vi "camMain - Copy.vi"() -> ()   [LabVIEW 2018]
uses:
  State control.ctl
  <vilib>/userdefined/High Color/IMAQdx.ctl
panel:
  out "Image":T1(plugin-control)
  in  "stop":bool
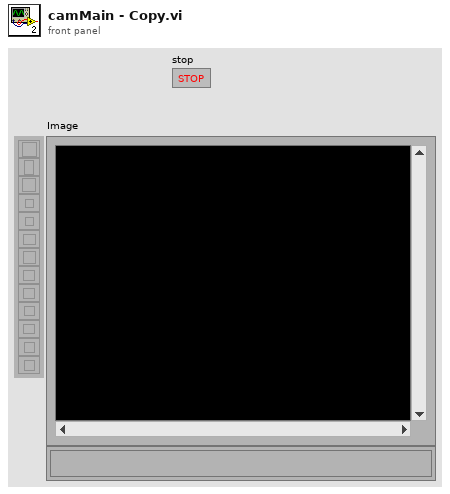
[diagram p1: front panel]
types:
  T1 = typedef "IMAQ Image.ctl" = refnum<image>
  T2 = typedef "IMAQdx.ctl" = refnum<k21>
  T3 = typedef "State control.ctl" = enum16{"Initialise", "Start camera", "Continuous Acquisition ", "Stop camera", "Dispose all"}
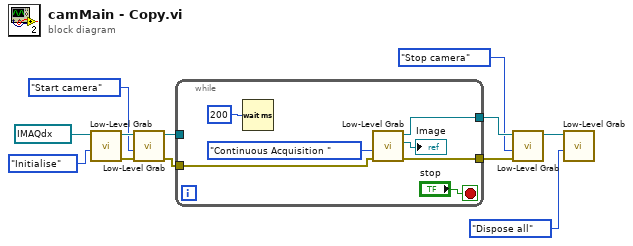
[diagram p0: block diagram]
diagram:
  n1 = call "Low-Level Grab.vi"("States"=State_control."Initialise", "Session In"=T2 "cam2") -> ("error out"=w9:errorcluster, "Session Out"=w10:T2)  [unwired: 7 in, 1 out]
  n2 = call "Low-Level Grab.vi"("error in (no error)"=w9, "States"=State_control."Start camera", "Session In"=w10) -> ("error out"=w1:errorcluster, "Session Out"=w7:T2)  [unwired: 6 in, 1 out]
  n3 = while {
    tunnel: w7 -> [_]
    tunnel: [w16] -> w6
    tunnel: [w15] -> w5
    tunnel: w1 -> [w13]
    stop <- "stop" stop-if-true
    n4 = Wait (ms)(milliseconds to wait=u32 200) -> ()  [unwired: 1 out]
    n5 = call "Low-Level Grab.vi"("error in (no error)"=w13, "States"=State_control."Continuous Acquisition ") -> ("error out"=w15:errorcluster, "Image Out"=→"Image":T1, "Session Out"=w16:T2)  [unwired: 7 in]
  }
  n6 = call "Low-Level Grab.vi"("error in (no error)"=w5, "States"=State_control."Stop camera", "Session In"=w6) -> ("Session Out"=w3:T2)  [unwired: 6 in, 2 out]
  n7 = call "Low-Level Grab.vi"("States"=State_control."Dispose all", "Session In"=w3) -> ()  [unwired: 7 in, 3 out]
